vi "DriveExecute.vi"(8 "error in (no error)":errorcluster) -> (0 "error out":errorcluster)   [LabVIEW 2023]
doc: "Execute for Drie\n\nClosed control loop for drive\n\ninput: \n error in (cluster)\n\noutput:\n error out (cluster)"
uses:
  DriveGlobal.vi
  <vilib>/Rock Robotics/WPI/ThirdParty/JAS_Junk/TrajLib/Trajectory_Library.lvlib
  <vilib>/Rock Robotics/WPI/ThirdParty/JAS_Junk/TrajLib/LinearFilter_LP_BW1_Execute.vi
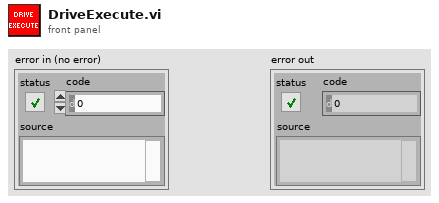
[diagram p1: front panel]
types:
  T1 = typedef "Trajectory_Library.lvlib/CHASSIS_SPEEDS.ctl" = cluster{"vX":dbl, "vY":dbl, "vOmega":dbl}
  T2 = typedef "ADIS16470 Device Reference.ctl" = cluster{"DevStatus":errorcluster, "Hardware Config":T3, "Calibration Complete":refnum<notifier>, "Status Reference":refnum<data-value>, "Data Reference":refnum<data-value>, "Sychronous Process VI":T7, "Cmd FIFO":refnum<k33>, "Source":T8, "Data FIFO":refnum<k33>, "Calibration Time (ms)":u32, "Data Reference":refnum<data-value>}
  T3 = typedef "ADIS16470 Hardware Configuration.ctl" = cluster{"SPI Clock Rate (Hz)":dbl, "IMU SPI Mode (3)":T4, "IMU Reset Pin":T5, "IMU SPI Bus":T6, "IMU Data Ready Pin":T5, "Stall Config":cluster{"Pow2BytesPerRead":u8, "StallTicks":u16, "CsToSclkTicks":u8}}
  T4 = typedef "WPI_SPIMode.ctl" = enum16{"Mode 0 (Clk Idle Low,Sample on Leading)", "Mode 1 (Clk Idle Low,Sample on Trailing)", "Mode 2 (Clk Idle High,Sample on Leading)", "Mode 3 (Clk Idle High,Sample on Trailing)"}
  T5 = typedef "FPGA_DIOChannel.ctl" = enum8{"DIO 0", "DIO 1", "DIO 2", "DIO 3", "DIO 4", "DIO 5", "DIO 6", "DIO 7", "DIO 8", "DIO 9", "DIO MXP 0", "DIO MXP 1", "DIO MXP 2", "DIO MXP 3", "DIO MXP 4", "DIO MXP 5", "DIO MXP 6", "DIO MXP 7", "DIO MXP 8", "DIO MXP 9", "DIO MXP 10", "DIO MXP 11", "DIO MXP 12", "DIO MXP 13", "DIO MXP 14", "DIO MXP 15", "SPI Port CS1", "SPI Port CS2", "SPI Port CS3", "SPI Port MISO", "SPI Port MOSI", "Invalid"}
  T6 = typedef "spi_bus.ctl" = enum16{"SPI On-Board, CS0", "SPI On-Board, CS1", "SPI On-Board, CS2", "SPI On-Board, CS3", "SPI MXP", "Invalid"}
  T7 = typedef "ADIS16470 Process.ctl" = refnum<vi>
  T8 = typedef "FPGA_CounterEncoderSourceConvertionLVSourceType.ctl" = cluster{"DevStatus":errorcluster, "AnalogTriggerMode?":bool, "DigitalMode":cluster{"DIO Channel":T9}, "AnalogTriggerMode":cluster{"AnalogTriggerIndex":T10, "OutputType":T11}}
  T9 = typedef "FPGA_DIODigitalSourceChannel.ctl" = enum8{"DIO 0", "DIO 1", "DIO 2", "DIO 3", "DIO 4", "DIO 5", "DIO 6", "DIO 7", "DIO 8", "DIO 9", "DIO MXP 0", "DIO MXP 1", "DIO MXP 2", "DIO MXP 3", "DIO MXP 4", "DIO MXP 5", "DIO MXP 6", "DIO MXP 7", "DIO MXP 8", "DIO MXP 9", "DIO MXP 10", "DIO MXP 11", "DIO MXP 12", "DIO MXP 13", "DIO MXP 14", "DIO MXP 15", "SPI Port CS1", "SPI Port CS2", "SPI Port CS3", "SPI Port MISO", "SPI Port MOSI", "Disabled"}
  T10 = typedef "FPGA_AnalogTriggerIndex.ctl" = enum8{"Trig 0", "Trig 1", "Trig 2", "Trig 3", "Trig 4", "Trig 5", "Trig 6", "Trig 7", "Invalid"}
  T11 = typedef "FPGA_AnalogTriggerOutType.ctl" = enum16{"InWindow", "TriggerState", "Rising", "Falling"}
  T12 = typedef "Trajectory_Library.lvlib/SWERVE_DRIVE_KINEMATICS.ctl" = cluster{"NumModules":i32, "InverseKinematics":T13, "ForwardKinematics":T13, "Modules":T14[], "PrevCoR":T14, "SavedModuleStates":T15[]}
  T13 = typedef "NI_Matrix.lvlib/RealMatrix.ctl" = dbl[][]
  T14 = typedef "Trajectory_Library.lvlib/TRANSLATION2D.ctl" = cluster{"X":dbl, "Y":dbl}
  T15 = typedef "Trajectory_Library.lvlib/SWERVE_DRIVE_MODULE_STATE.ctl" = cluster{"Speed":dbl, "Angle":T16}
  T16 = typedef "Trajectory_Library.lvlib/ROTATION2D.ctl" = cluster{"VALUE":dbl, "COS":dbl, "SIN":dbl}
  T17 = typedef "Trajectory_Library.lvlib/SWERVE_DRIVE_MODULE_POSITION.ctl" = cluster{"Distance":dbl, "Angle":T16, "P":bool}
  T18 = typedef "ADIS16470 Data.ctl" = cluster{"XAngle":dbl, "YAngle":dbl, "ZAngle":dbl}
  T19 = typedef "ADIS16470 Status.ctl" = cluster{"Calibrated?":bool, "IMU Detected?":bool}
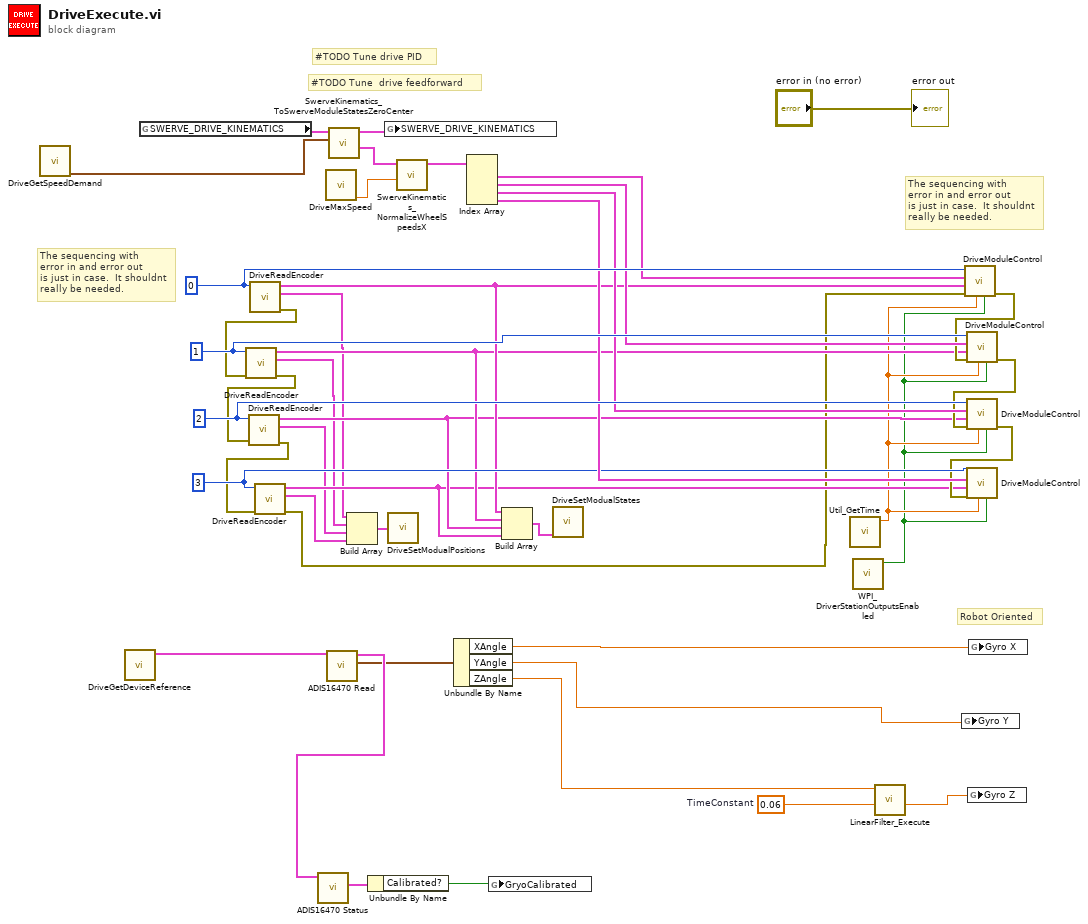
[diagram p0: block diagram]
diagram:
  w3 = 0.06  # TimeConstant
  w40 = 0 ("ModualNamePrefix")
  w39 = 1 ("ModualNamePrefix")
  w38 = 2 ("ModualNamePrefix")
  w33 = 3 ("ModualNamePrefix")
  # "#TODO Tune drive PID"
  # "#TODO Tune  drive feedforward"
  # "Robot Oriented"
  # "The sequencing with\nerror in and error out\nis just in case.  It shouldnt\nreally be needed."
  # "The sequencing with\nerror in and error out\nis just in case.  It shouldnt\nreally be needed."
  n1 = call "DriveGetSpeedDemand.vi"() -> ("ChassisSpeedDemand"=w42:T1)  [unwired: 8 in, 3 out]
  n2 = call "DriveGetDeviceReference.vi"() -> ("ADIS16470DevRef out"=w16:T2)  [unwired: 11 in]
  n3 = global read "DriveGlobal.vi" "SWERVE_DRIVE_KINEMATICS"() -> (w43:T12)
  n4 = call "DriveReadEncoder.vi"("ModualNamePrefix"=w40) -> ("error out"=w19:errorcluster, "SWERVE_DRIVE_MODULE_POSITION"=w25:T17, "SWERVE_DRIVE_MODULE_STATE"=w29:T15)  [unwired: 8 in]
  n5 = call "DriveReadEncoder.vi"("error in"=w19, "ModualNamePrefix"=w39) -> ("error out"=w18:errorcluster, "SWERVE_DRIVE_MODULE_POSITION"=w24:T17, "SWERVE_DRIVE_MODULE_STATE"=w28:T15)  [unwired: 7 in]
  n6 = call "DriveReadEncoder.vi"("error in"=w18, "ModualNamePrefix"=w38) -> ("error out"=w17:errorcluster, "SWERVE_DRIVE_MODULE_POSITION"=w23:T17, "SWERVE_DRIVE_MODULE_STATE"=w27:T15)  [unwired: 7 in]
  n7 = call "DriveReadEncoder.vi"("error in"=w17, "ModualNamePrefix"=w33) -> ("error out"=w7:errorcluster, "SWERVE_DRIVE_MODULE_POSITION"=w22:T17, "SWERVE_DRIVE_MODULE_STATE"=w26:T15)  [unwired: 7 in]
  n8 = call "DriveMaxSpeed.vi"() -> ("Max Speed (m/sec)"=w5:dbl)  [unwired: 10 in, 1 out]
  n9 = call <vilib>:"ADIS16470 Read.vi"("ADIS16470DevRef"=w16) -> ("ADIS16470 Value"=w12:T18, "ADIS16470DevRef"=w13:T2)  [unwired: 7 in, 2 out]
  n10 = call <vilib>:"ADIS16470 Status.vi"("ADIS16470DevRef"=w13) -> ("ADIS16470 Status"=w15:T19)  [unwired: 8 in, 2 out]
  n11 = call <vilib>:"SwerveKinematics_ToSwerveModuleStatesZeroCenter.vi"("ChassisSpeeds"=w42, "in SWERVE_DRIVE_KINEMATICS"=w43) -> ("ModuleStates"=w6:T15[], "out SWERVE_DRIVE_KINEMATICS"=w41:T12)  [unwired: 8 in]
  n12 = Build Array(w25, w24, w23, w22) -> (w20:T17[])
  n13 = Unbundle By Name(w15) -> ("Calibrated?"=w14:bool)
  n14 = global write "DriveGlobal.vi" "SWERVE_DRIVE_KINEMATICS"(w41) -> ()
  n15 = call "DriveSetModualPositions.vi"("Swerve_Drive_Modual_Position"=w20) -> ()  [unwired: 11 in]
  n16 = call <vilib>:"SwerveKinematics_NormalizeWheelSpeedsX.vi"("AttainableMaxSpeed"=w5, "in WheelStates"=w6) -> ("out WheelStates"=w4:T15[])  [unwired: 9 in]
  n17 = Unbundle By Name(w12) -> ("XAngle"=w10:dbl, "YAngle"=w9:dbl, "ZAngle"=w11:dbl)
  n18 = Index Array(array=w4) -> (element #1=w34:T15, element #2=w37:T15, element #3=w36:T15, element #4=w35:T15)  [unwired: 4 in]
  n19 = global write "DriveGlobal.vi" "GryoCalibrated"(w14) -> ()
  n20 = Build Array(w29, w28, w27, w26) -> (w21:T15[])
  n21 = call "DriveSetModualStates.vi"("Swerve__Drive_Modual_States"=w21) -> ()  [unwired: 11 in]
  n22 = call <vilib>:"Util_GetTime.vi"() -> ("FPGA_Time_Seconds"=w2:dbl)  [unwired: 9 in, 2 out]
  n23 = call <vilib>:"WPI_DriverStationOutputsEnabled.vi"() -> ("OutputsEnabled?"=w1:bool)  [unwired: 10 in, 1 out]
  n24 = call-poly <vilib>:"LinearFilter_Execute.vi"("TimeConstant"=w3, "Input"=w11) -> ("Output"=w8:dbl)  [unwired: 9 in]
  n25 = global write "DriveGlobal.vi" "Gyro Y"(w9) -> ()
  n26 = call "DriveModuleControl.vi"("Outputs Enabled"=w1, "Pass Through Time"=w2, "error in"=w7, "Actual State"=w29, "Desired State"=w34, "ModuleIndex"=w40) -> ("error out"=w32:errorcluster)  [unwired: 5 in]
  n27 = call "DriveModuleControl.vi"("Outputs Enabled"=w1, "Pass Through Time"=w2, "error in"=w32, "Actual State"=w28, "Desired State"=w37, "ModuleIndex"=w39) -> ("error out"=w31:errorcluster)  [unwired: 5 in]
  n28 = call "DriveModuleControl.vi"("Outputs Enabled"=w1, "Pass Through Time"=w2, "error in"=w31, "Actual State"=w27, "Desired State"=w36, "ModuleIndex"=w38) -> ("error out"=w30:errorcluster)  [unwired: 5 in]
  n29 = call "DriveModuleControl.vi"("Outputs Enabled"=w1, "Pass Through Time"=w2, "error in"=w30, "Actual State"=w26, "Desired State"=w35, "ModuleIndex"=w33) -> ()  [unwired: 5 in, 1 out]
  n30 = global write "DriveGlobal.vi" "Gyro Z"(w8) -> ()
  n31 = global write "DriveGlobal.vi" "Gyro X"(w10) -> ()
  "error out" <- "error in (no error)"
